vi "Assert String Contains String Ignoring Case.vi"(5 "Needle":string, 7 "Message (\"\")":string, 8 "error in (no error)":errorcluster, 10 "Haystack":string) -> (0 "error out":errorcluster)   [LabVIEW 2017, in "Transparent Assertions.lvlib" / "Assertions.lvlib"]
doc: "Asserts that a string contains the expected substring, ignoring case differences. Returns an error if the assertion fails, and optionally appends a custom message to the error."
uses:
  Assertions.lvlib
  Constraints/StringContains/StringContains.lvclass
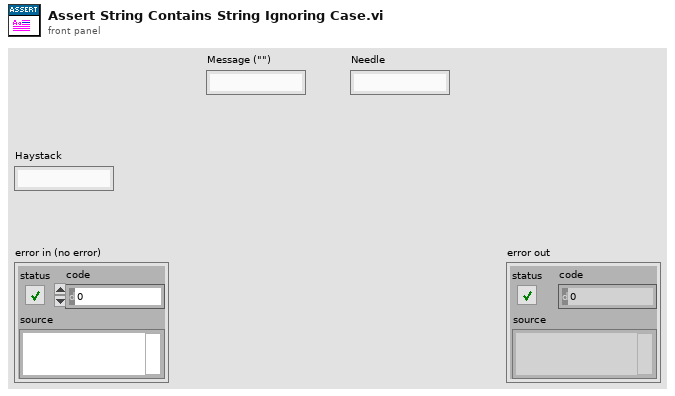
[diagram p1: front panel]
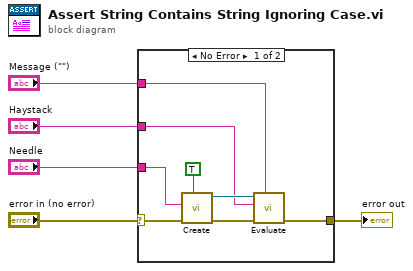
[diagram p0: block diagram]
diagram:
  n1 = case shown="No Error" "error in (no error)" {
    selector: "error in (no error)" -> [w8 w14]
    tunnel: "Haystack" -> [w11 _]
    tunnel: [w10 w14] -> w4
    tunnel: "Message (\"\")" -> [w9 _]
    tunnel: "Needle" -> [w7 _]
    frame No Error {
      n2 = call "Create.vi"("Ignore Case (F)"=TRUE, "error in (no error)"=w8, "Needle"=w7) -> ("error out"=w12:errorcluster, "StringContains"=w13:refnum<class "StringContains.lvclass">)  [unwired: 7 in]
      n3 = call-dynamic "Evaluate.vi"("Message (\"\")"=w9, "error in (no error)"=w12, "Actual"=w11, "Constraint in"=w13) -> ("error out"=w10:errorcluster)  [unwired: 6 in, 1 out]
    }
    frame Error {
    }
  }
  "error out" <- w4
